vi "Initalize.vi"(8 "error in (no error)":errorcluster, 9 "Section":string, 10 "Config Path":path, 11 "SIM Motion Controller in":refnum<class "SIM Motion Controller.lvclass">) -> (0 "error out":errorcluster, 3 "SIM Motion Controller out":refnum<class "SIM Motion Controller.lvclass">)   [LabVIEW 2022 SP3, in "SIM Motion Controller.lvclass"]
uses:
  SIM Motion Controller.lvclass
  C:/Users/Josh.Thibeault/Desktop/MAS/Base/Base.lvclass
  Base/Base.lvclass/Base.ctl
  Base/Accessors/Write Config Path.vi
  Base/Accessors/Write Section.vi
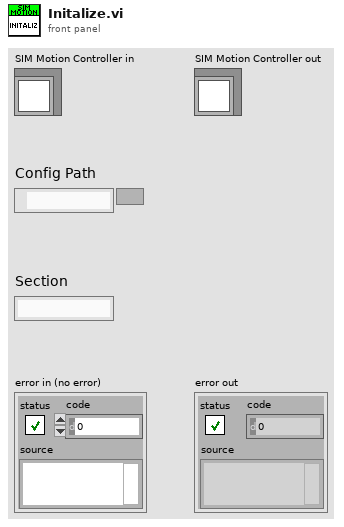
[diagram p1: front panel]
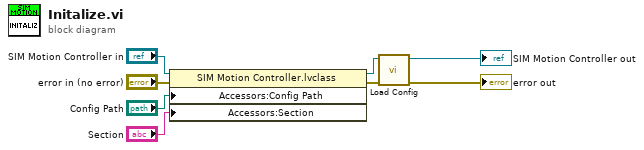
[diagram p0: block diagram]
diagram:
  n1 = property class="SIM Motion Controller.lvclass"(reference="SIM Motion Controller in", error in="error in (no error)", "Accessors:Config Path"="Config Path", "Accessors:Section"="Section") -> (reference out=w6:refnum<class "SIM Motion Controller.lvclass">, error out=w2:errorcluster)
  n2 = call-dynamic "Load Config.vi"("error in (no error)"=w2, "SIM Motion Controller in"=w6) -> ("error out"=→"error out":errorcluster, "SIM Motion Controller out"=→"SIM Motion Controller out":refnum<class "SIM Motion Controller.lvclass">)  [unwired: 8 in]
